vi "ATDome_getEvent_scbLink.vi"(8 "error in (no error)":errorcluster, 11 "logevent_scbLink_Ctl":T1) -> (0 "error out":errorcluster, 2 "function return":i32, 3 "logevent_scbLink_Ctl out":T1)   [LabVIEW 2016, in "SALLV_ATDome.lvlib"]
doc: "int ATDome_shm_getEvent_scbLinkLV(ATDome_logevent_scbLinkLV *logevent_scbLink_Ctl );"
uses:
  SALLV_ATDome.lvlib
  DataTypes/logevent_scbLink.ctl
  SALLV_ATDome.so
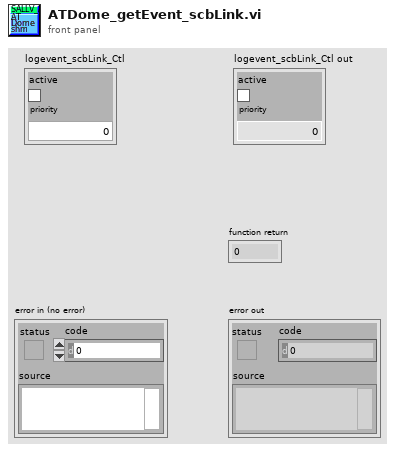
[diagram p1: front panel]
types:
  T1 = typedef "SALLV_ATDome.lvlib/logevent_scbLink.ctl" = cluster{"active":bool, "priority":i32}
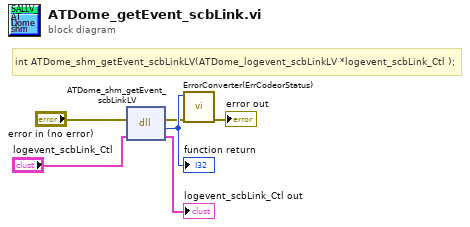
[diagram p0: block diagram]
diagram:
  # "int ATDome_shm_getEvent_scbLinkLV(ATDome_logevent_scbLinkLV *logevent_scbLink_Ctl );"
  n1 = dll-call lib="home/andres/Desktop/SAL_ATDome/SALLV_ATDome.*" fn="ATDome_shm_getEvent_scbLinkLV"(error in="error in (no error)", "logevent_scbLink_Ctl"="logevent_scbLink_Ctl") -> (error out=w2:errorcluster, w6:i32, "logevent_scbLink_Ctl"=→"logevent_scbLink_Ctl out":T1)  [unwired: 2 in, 1 out]
  "function return" <- w6
  n2 = call "ErrorConverter(ErrCodeorStatus).vi"("error in (no error)"=w2, "error code"=w6) -> ("error out"=→"error out":errorcluster)  [unwired: 9 in]
